vi "GetURL.vi"(11 "IDs":T1) -> (3 "String":string)   [LabVIEW 2022 SP3]
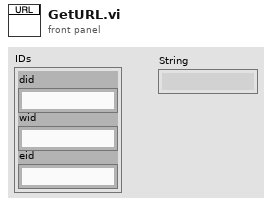
[diagram p1: front panel]
types:
  T1 = cluster{"did":string, "wid":string, "eid":string}
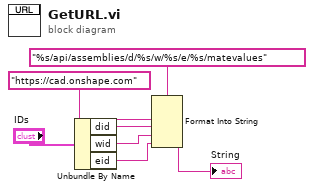
[diagram p0: block diagram]
diagram:
  n1 = Unbundle By Name("IDs") -> ("did"=w1:string, "wid"=w4:string, "eid"=w5:string)
  n2 = Format Into String(format string="%s/api/assemblies/d/%s/w/%s/e/%s/matevalues" ("payload"), "https://cad.onshape.com" ("stacks"), w1, w4, w5) -> (resulting string=→"String":string)  [unwired: 2 in, 1 out]
